vi "ReadAndWrite.vi"(7 "Enum":enum16{"initial", "save", "read"}(ring)=enum."save", 8 "error in":errorcluster, 11 "Tab Control":refnum<vi>) -> (0 "error out":errorcluster)   [LabVIEW 2019]
uses:
  Ctrl/ProjectSetAction.ctl
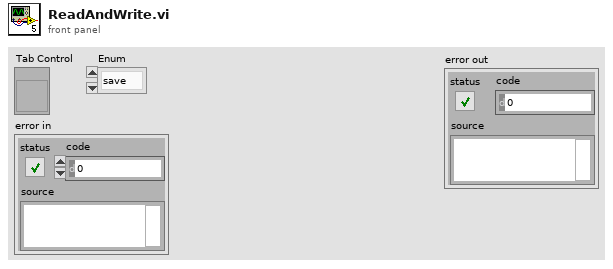
[diagram p1: front panel]
types:
  T1 = typedef "ProjectSetAction.ctl" = enum16{"initial", "save", "load", "write", "read"}
  T2 = enum16{"initial", "save", "load", "write", "read"}
  T3 = cluster{"type string":i16[], "data string":string}
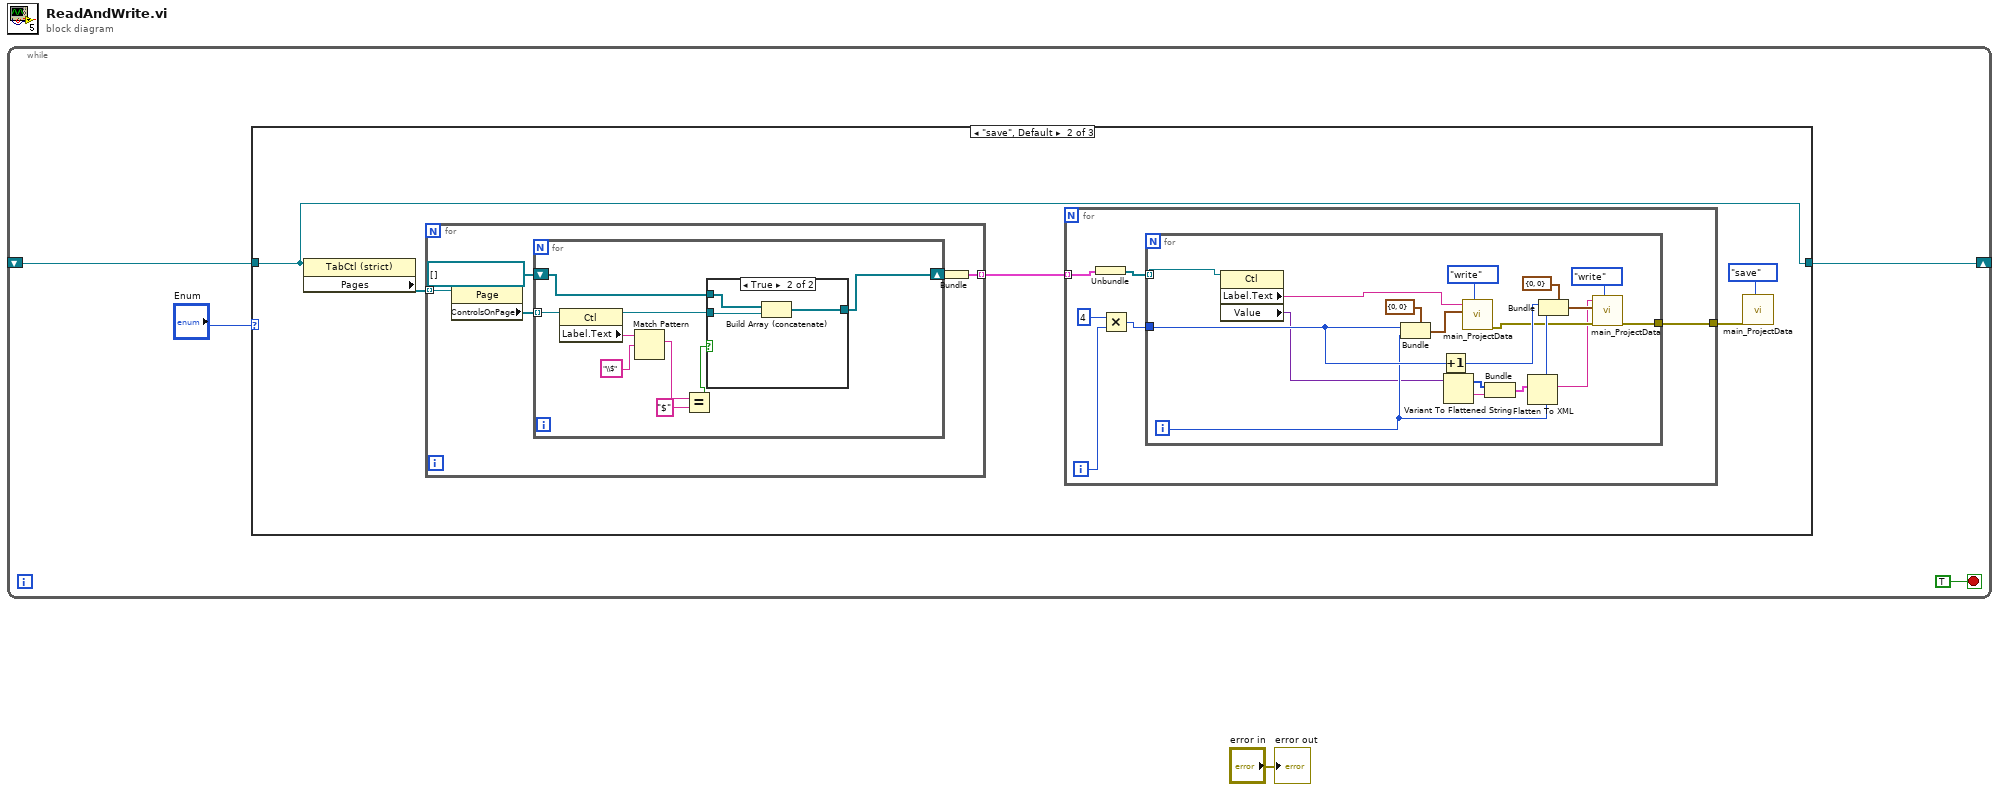
[diagram p0: block diagram]
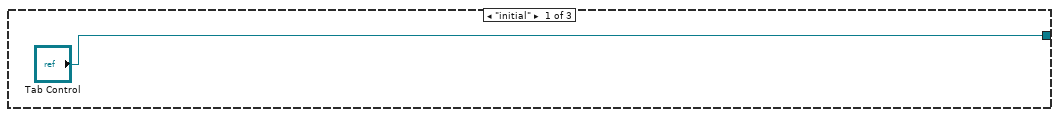
[diagram p2: hidden frame]
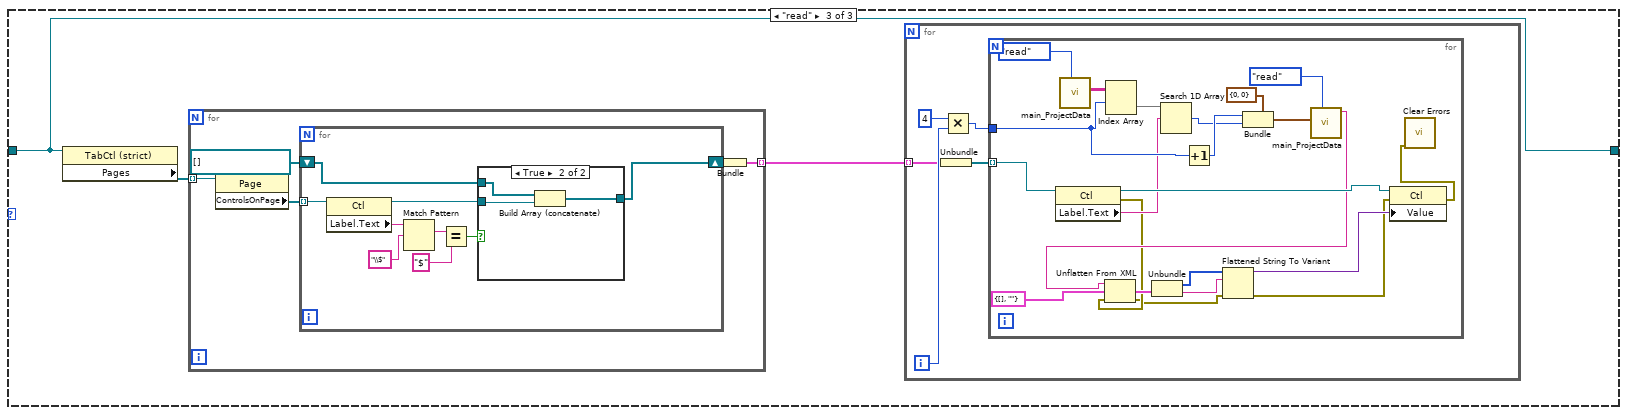
[diagram p4: hidden frame]
diagram:
  n1 = while {
    shift-right: [w2] -> _
    shift-left: _ -> [w5]
    stop <- TRUE stop-if-true
    n2 = case shown="\"save\", Default" "Enum" {
      tunnel: w5 -> [_ w9 w54]
      tunnel: ["Tab Control" w9 w54] -> w2
      frame "initial" {
      }
      frame "save", Default {
        n3 = property class="TabCtl (strict)"(reference=w9) -> ("Pages"=w11:refnum<vi>[])  [unwired: 1 in, 2 out]
        n4 = for {
          tunnel: w11 -> [w40] mode=indexing
          tunnel: [w36] -> w10 mode=indexing
          n5 = property class="Page"(reference=w40) -> ("ControlsOnPage"=w39:refnum<vi>[])  [unwired: 1 in, 2 out]
          n6 = for {
            tunnel: w39 -> [w49] mode=indexing
            shift-right: [w45] -> w37
            shift-left: refnum<vi>[] [] -> [w44]
            n7 = property class="Ctl"(reference=w49) -> (reference out=w46:refnum<vi>, "Label.Text"=w48:string)  [unwired: 1 in, 1 out]
            n8 = Match Pattern(string=w48, regular expression="\\$") -> (match substring=w43:string)  [unwired: 1 in, 3 out]
            n9 = Equal?(x=w43, y="$") -> (x = y?=w41:bool)
            n10 = case shown="True" w41 {
              tunnel: w46 -> [_ w53]
              tunnel: [w50 w52] -> w45
              tunnel: w44 -> [w50 w51]
              frame False {
              }
              frame True {
                n11 = Build Array (concatenate)(w51, w53) -> (w52:refnum<vi>[])
              }
            }
          }
          n12 = Bundle(w37) -> (w36:cluster{refnum<vi>[]})  [unwired: 1 in]
        }
        n13 = for {
          tunnel: w10 -> [w14] mode=indexing
          tunnel: [w12] -> w8
          i -> [w17]
          n14 = Unbundle(w14) -> (w13:refnum<vi>[])
          n15 = Multiply(x=4, y=w17) -> (x*y=w15:i32)
          n16 = for {
            tunnel: w15 -> [w32]
            tunnel: w13 -> [w26] mode=indexing
            tunnel: [w25] -> w12
            i -> [w29]
            n17 = property class="Ctl"(reference=w26) -> ("Label.Text"=w33:string, "Value"=w24:variant)  [unwired: 1 in, 2 out]
            n18 = Bundle(cluster=cluster{"Y":i32, "X":i32} {"Y"=0, "X"=0} ("Index"), "Y"=w32, "X"=w29) -> (w34:cluster{"Y":i32, "X":i32})
            n19 = Increment(x=w32) -> (x+1=w30:i32)
            n20 = Variant To Flattened String(Variant=w24) -> (data string=w22:string, 1:w23:i16[])
            n21 = call "main_ProjectData.vi"("Enum"=ProjectSetAction."write", "Index"=w34, "DataIn"=w33) -> ("error out"=w27:errorcluster)  [unwired: 6 in, 2 out]
            n22 = Bundle("type string"=w23, "data string"=w22) -> (w21:T3)  [unwired: 1 in]
            n23 = Flatten To XML(anything=w21) -> (xml string=w20:string)
            n24 = Bundle(cluster=cluster{"Y":i32, "X":i32} {"Y"=0, "X"=0} ("Index"), "Y"=w30, "X"=w29) -> (w28:cluster{"Y":i32, "X":i32})
            n25 = call "main_ProjectData.vi"("Enum"=ProjectSetAction."write", "error in"=w27, "Index"=w28, "DataIn"=w20) -> ("error out"=w25:errorcluster)  [unwired: 5 in, 2 out]
          }
        }
        n26 = call "main_ProjectData.vi"("Enum"=ProjectSetAction."save", "error in"=w8) -> ()  [unwired: 7 in, 3 out]
      }
      frame "read" {
        n27 = property class="TabCtl (strict)"(reference=w54) -> ("Pages"=w56:refnum<vi>[])  [unwired: 1 in, 2 out]
        n28 = for {
          tunnel: w56 -> [w88] mode=indexing
          tunnel: [w84] -> w55 mode=indexing
          n29 = property class="Page"(reference=w88) -> ("ControlsOnPage"=w87:refnum<vi>[])  [unwired: 1 in, 2 out]
          n30 = for {
            tunnel: w87 -> [w97] mode=indexing
            shift-right: [w91] -> w85
            shift-left: refnum<vi>[] [] -> [w90]
            n31 = property class="Ctl"(reference=w97) -> (reference out=w92:refnum<vi>, "Label.Text"=w96:string)  [unwired: 1 in, 1 out]
            n32 = Match Pattern(string=w96, regular expression="\\$") -> (match substring=w95:string)  [unwired: 1 in, 3 out]
            n33 = Equal?(x=w95, y="$") -> (x = y?=w93:bool)
            n34 = case shown="True" w93 {
              tunnel: w92 -> [_ w101]
              tunnel: [w98 w100] -> w91
              tunnel: w90 -> [w98 w99]
              frame False {
              }
              frame True {
                n35 = Build Array (concatenate)(w99, w101) -> (w100:refnum<vi>[])
              }
            }
          }
          n36 = Bundle(w85) -> (w84:cluster{refnum<vi>[]})  [unwired: 1 in]
        }
        n37 = for {
          tunnel: w55 -> [w60] mode=indexing
          i -> [w61]
          n38 = Unbundle(w60) -> (w57:refnum<vi>[])
          n39 = Multiply(x=4, y=w61) -> (x*y=w58:i32)
          n40 = for {
            tunnel: w58 -> [w80]
            tunnel: w57 -> [w83] mode=indexing
            n41 = property class="Ctl"(reference=w83) -> (reference out=w75:refnum<vi>, error out=w65:errorcluster, "Label.Text"=w74:string)  [unwired: 1 in]
            n42 = call "main_ProjectData.vi"("Enum"=T2."read") -> ("Table Control"=w82:string[][])  [unwired: 8 in, 2 out]
            n43 = Index Array(array=w82, index (row)=w80) -> (element=w81:string[])  [unwired: 1 in]
            n44 = Search 1D Array(1D array=w81, element=w74) -> (index of element=w77:i32)  [unwired: 1 in]
            n45 = Increment(x=w80) -> (x+1=w78:i32)
            n46 = Bundle(cluster=cluster{"Y":i32, "X":i32} {"Y"=0, "X"=0} ("Index"), "Y"=w78, "X"=w77) -> (w76:cluster{"Y":i32, "X":i32})
            n47 = call "main_ProjectData.vi"("Enum"=ProjectSetAction."read", "Index"=w76) -> ("DataOut"=w73:string)  [unwired: 7 in, 2 out]
            n48 = Unflatten From XML(xml string=w73, type=T3 {"type string"=[], "data string"=""} ("cluster"), error in (no error)=w65) -> (value=w71:T3, error out=w64:errorcluster)
            n49 = Unbundle(w71) -> ("type string"=w70:i16[], "data string"=w69:string)
            n50 = Flattened String To Variant(4:w64, 6:w69, 7:w70) -> (0:w67:errorcluster, 3:w68:variant)
            n51 = property class="Ctl"(reference=w75, error in=w67, "Value"=w68) -> (error out=w66:errorcluster)  [unwired: 1 out]
            n52 = call <vilib>:"Clear Errors.vi"("error in (no error)"=w66) -> ()  [unwired: 5 in, 2 out]
          }
        }
      }
    }
  }
  "error out" <- "error in"
